vi "_[error50000]Invalid DB REF.vi"(6 "Force Gen?":bool, 8 "error in (no error)":errorcluster) -> (0 "error out":errorcluster)   [LabVIEW 2017, in "TagDB.lvlib"]
uses:
  TagDB.lvlib
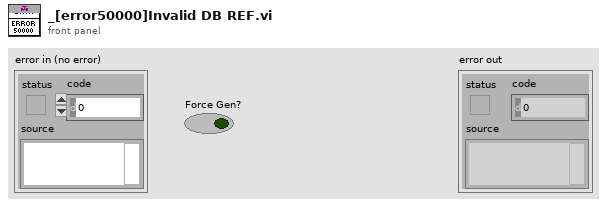
[diagram p1: front panel]
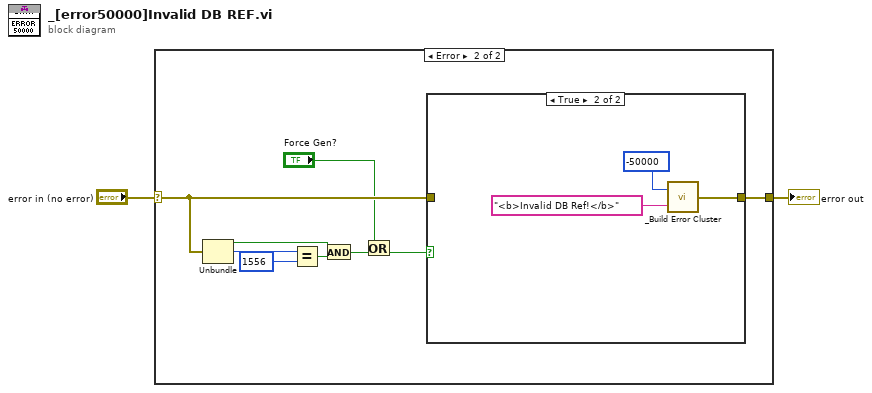
[diagram p0: block diagram]
diagram:
  n1 = case shown="Error" "error in (no error)" {
    selector: "error in (no error)" -> [w3 w11]
    tunnel: [w3 w12] -> w2
    frame No Error {
    }
    frame Error {
      n2 = Unbundle(w11) -> ("status"=w6:bool, "code"=w10:i32)  [unwired: 1 out]
      n3 = Equal?(x=w10, y=1556) -> (x = y?=w8:bool)
      n4 = And(x=w6, y=w8) -> (x .and. y?=w7:bool)
      n5 = Or(x="Force Gen?", y=w7) -> (x .or. y?=w5:bool)
      n6 = case shown="True" w5 {
        tunnel: [w13 w14] -> w12
        tunnel: w11 -> [w13 _]
        frame False {
        }
        frame True {
          n7 = call "_Build Error Cluster.vi"("String to Prepend to source (\"\")"="<b>Invalid DB Ref!</b>" ("source"), "code"=-50000) -> ("error out"=w14:errorcluster)
        }
      }
    }
  }
  "error out" <- w2
